vi "ColorGlobals.vi"() -> ()   [LabVIEW 2020]
panel:
  in  "Line numbers":u32(colorbox)=16300287
  in  "REPL Error":u32(colorbox)=15665920
  in  "REPL Text":u32(colorbox)=16448250
  in  "FIFO":i32=10000
  in  "Python words":string[](array[string])=["False", "None", "True", "and", "as", "assert", "break", "class", "continue", "def", "del", "elif", "else", "except", "finally", "for", "from", "global", "if", "import", "in", "is", "lambda", "nonlocal", "not", "or", "pass", "raise", "return", "try", "while", "with", "yield", "print"]
  in  "Text":u32(colorbox)=16448250
  in  "Triple Quote":u32(colorbox)=9306312
  in  "Comment":u32(colorbox)=15665920
  in  "Python":u32(colorbox)=14453248
  in  "function":u32(colorbox)=239
  in  "Quote":u32(colorbox)=46086
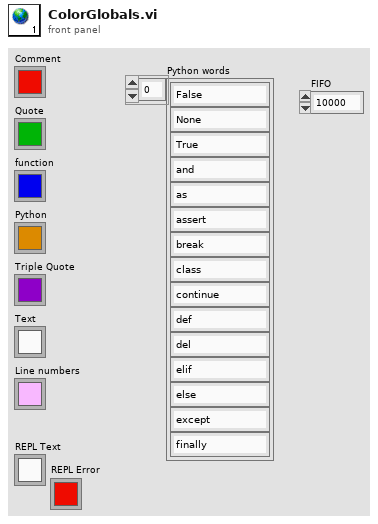
[diagram p1: front panel]
diagram:
